vi "Construct String.vi"(8 "error in (no error)":errorcluster, 10 "String":string) -> (0 "error out":errorcluster, 3 "String out":refnum<class "String.lvclass">)   [LabVIEW 2017, in "Composition.Tests.lvlib" / "String.lvclass"]
uses:
  String.lvclass
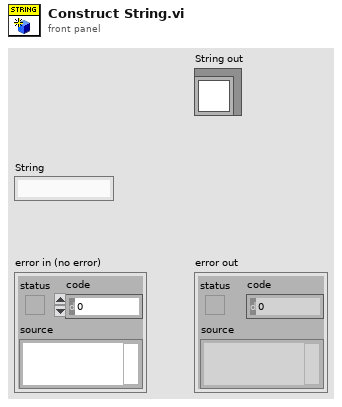
[diagram p1: front panel]
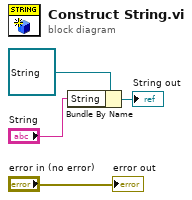
[diagram p0: block diagram]
diagram:
  n1 = Bundle By Name(cluster=refnum<class "String.lvclass"> refnum ("String in"), "String"="String") -> (→"String out":refnum<class "String.lvclass">)
  "error out" <- "error in (no error)"
